vi "MinMax.vi"(11 "2D Double Array":i32[][](array[numeric])) -> (0 "max in row":i32[](array[numeric]), 3 "min in row":i32[](array[numeric]))   [LabVIEW 2023]
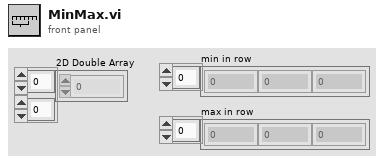
[diagram p1: front panel]
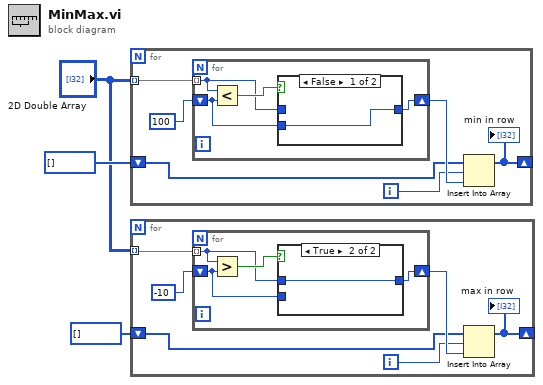
[diagram p0: block diagram]
diagram:
  n1 = for {
    tunnel: "2D Double Array" -> [w9] mode=indexing
    shift-right: [w5] -> _
    shift-left: i32[] [] -> [w4]
    i -> [w6]
    n2 = for {
      tunnel: w9 -> [w12] mode=indexing
      shift-right: [w11] -> w7
      shift-left: 100 ("element") -> [w10]
      n3 = Less?(x=w12, y=w10) -> (x < y?=w13:bool)
      n4 = case shown="False" w13 {
        tunnel: w12 -> [_ w15]
        tunnel: [w14 w15] -> w11
        tunnel: w10 -> [w14 _]
        frame False {
        }
        frame True {
        }
      }
    }
    n5 = Insert Into Array(array=w4, index=w6, new element=w7) -> (w5:i32[])
    "min in row" <- w5
  }
  n6 = for {
    tunnel: "2D Double Array" -> [w21] mode=indexing
    shift-right: [w17] -> _
    shift-left: i32[] [] -> [w16]
    i -> [w18]
    n7 = for {
      tunnel: w21 -> [w24] mode=indexing
      shift-right: [w23] -> w19
      shift-left: -10 ("element") -> [w22]
      n8 = Greater?(x=w24, y=w22) -> (0:w25:bool)
      n9 = case shown="True" w25 {
        tunnel: w24 -> [_ w27]
        tunnel: [w26 w27] -> w23
        tunnel: w22 -> [w26 _]
        frame False {
        }
        frame True {
        }
      }
    }
    n10 = Insert Into Array(array=w16, index=w18, new element=w19) -> (w17:i32[])
    "max in row" <- w17
  }
